vi "PID Stuff.vi"() -> ()   [LabVIEW 2023]
uses:
  MHZLib/Variables and Definitions/Auto_Values.ctl
  <vilib>/addons/control/pid/NI_PID_pid.lvlib
  <vilib>/addons/control/pid/pid.llb/PID (DBL).vi
panel:
  out "Rot Out":dbl format="%.2f"
  out "Y Out":dbl format="%.2f"
  out "X Out":dbl format="%.2f"
  in  "Auto Values":T1 {"Shooter Throttle" min=-360.0 max=360.0; "Rotation Tol (Deg)" min=-360.0 max=360.0; "Strafe Throttle" min=0.0 max=1.0}
  in  "PID x":T2={"proportional gain (Kc)"=1.0, "integral time (Ti, min)"=0.01, "derivative time (Td, min)"=0.0} {"derivative time (Td, min)" format="%.3f"; "integral time (Ti, min)" format="%.3f"; "proportional gain (Kc)" format="%.3f"}
  in  "PID y":T2={"proportional gain (Kc)"=1.0, "integral time (Ti, min)"=0.01, "derivative time (Td, min)"=0.0} {"derivative time (Td, min)" format="%.3f"; "integral time (Ti, min)" format="%.3f"; "proportional gain (Kc)" format="%.3f"}
  in  "PID rot":T2={"proportional gain (Kc)"=1.0, "integral time (Ti, min)"=0.01, "derivative time (Td, min)"=0.0} {"derivative time (Td, min)" format="%.3f"; "integral time (Ti, min)" format="%.3f"; "proportional gain (Kc)" format="%.3f"}
  in  "Target Rot":dbl
  in  "Target Y":dbl
  in  "Target X":dbl
  in  "Cancel":bool
  in  "Rotate Tolerance":dbl
  in  "Strafe Tolerance":dbl
  # "Takes precedence\nfrom Tol"
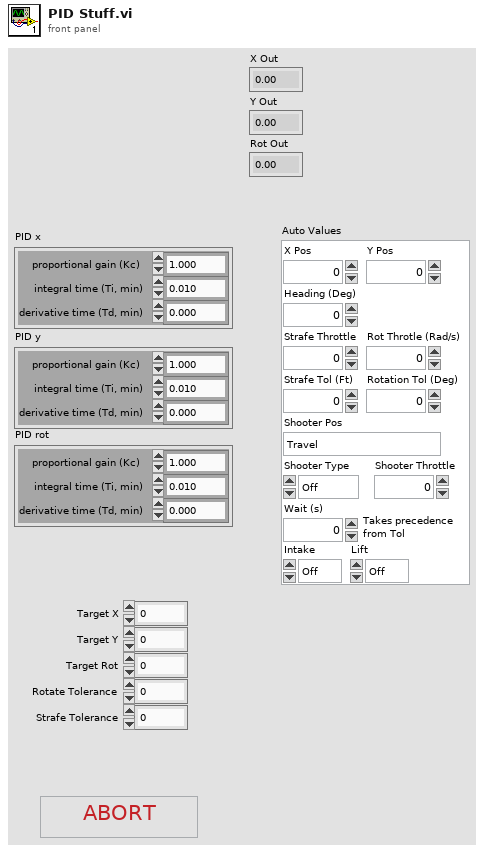
[diagram p1: front panel]
types:
  T1 = typedef "Auto_Values.ctl" = cluster{"X Pos":dbl, "Y Pos":dbl, "Heading (Deg)":dbl, "Strafe Throttle":dbl, "Rot Throtle (Rad/s)":dbl, "Strafe Tol (Ft)":dbl, "Rotation Tol (Deg)":dbl, "Shooter Pos":enum16{"Travel", "Speaker", "Amp"}, "Intake":enum16{"Off", "Front", "Center", "Out"}, "Shooter Type":enum16{"Off", "Manual", "Automatic"}, "Shooter Throttle":dbl, "Wait (s)":dbl, "Lift":enum16{"Off", "Up", "Down"}}
  T2 = cluster{"proportional gain (Kc)":dbl, "integral time (Ti, min)":dbl, "derivative time (Td, min)":dbl}
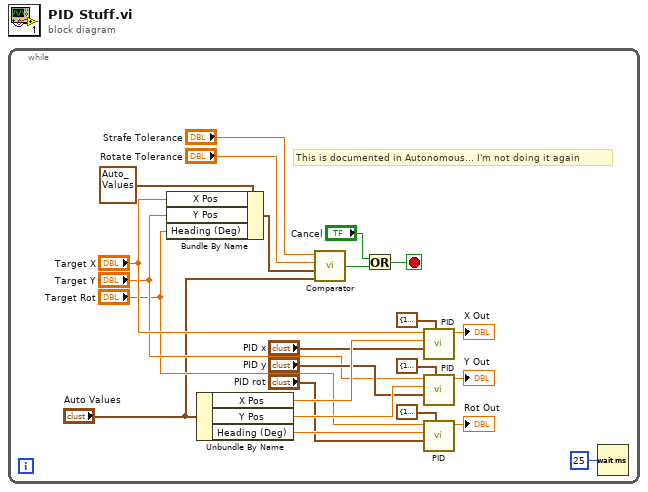
[diagram p0: block diagram]
diagram:
  n1 = while {
    stop <- w7 stop-if-true
    # "This is documented in Autonomous... I'm not doing it again"
    n2 = Bundle By Name(cluster=T1 {"X Pos"=0.0, "Y Pos"=0.0, "Heading (Deg)"=0.0, "Strafe Throttle"=0.0, "Rot Throtle (Rad/s)"=0.0, "Strafe Tol (Ft)"=0.0, "Rotation Tol (Deg)"=0.0, "Shooter Pos"=enum."Travel", "Intake"=enum."Front", "Shooter Type"=enum."Manual", "Shooter Throttle"=0.0, "Wait (s)"=0.0, "Lift"=enum."Off"} ("element"), "X Pos"="Target X", "Y Pos"="Target Y", "Heading (Deg)"="Target Rot") -> (w10:T1)
    n3 = Unbundle By Name("Auto Values") -> ("X Pos"=w20:dbl, "Y Pos"=w19:dbl, "Heading (Deg)"=w18:dbl)
    n4 = call "Comparator.vi"("Current Location"="Auto Values", "Target Location"=w10, "Rotate Tolerance"="Rotate Tolerance", "Strafe Tolerance"="Strafe Tolerance") -> ("In range?"=w9:bool)
    n5 = Or(x="Cancel", y=w9) -> (x .or. y?=w7:bool)
    n6 = call-poly <vilib>:"PID.vi"("output range"=cluster{"output high":dbl, "output low":dbl} {"output high"=1.0, "output low"=-1.0}, "PID gains"="PID x", "process variable"=w20, "setpoint"="Target X") -> ("output"=→"X Out":dbl)  [unwired: 6 in, 1 out]
    n7 = call-poly <vilib>:"PID.vi"("output range"=cluster{"output high":dbl, "output low":dbl} {"output high"=1.0, "output low"=-1.0}, "PID gains"="PID y", "process variable"=w19, "setpoint"="Target Y") -> ("output"=→"Y Out":dbl)  [unwired: 6 in, 1 out]
    n8 = call-poly <vilib>:"PID.vi"("output range"=cluster{"output high":dbl, "output low":dbl} {"output high"=1.0, "output low"=-1.0}, "PID gains"="PID rot", "process variable"=w18, "setpoint"="Target Rot") -> ("output"=→"Rot Out":dbl)  [unwired: 6 in, 1 out]
    n9 = Wait (ms)(milliseconds to wait=u32 25) -> ()  [unwired: 1 out]
  }
